vi "Run_Command.vi"(0 "Event":cluster{string, string[], dbl[], dbl}, 1 "Debug Mode":bool, 2 "Realtime Debug":bool, 3 "Update Functions In":cluster{string, string[], dbl[], dbl}[](array[cluster]), 4 "API Function Array":cluster{string, "VI Reference":refnum<vi>}[](array[cluster])) -> (5 "Update Functions Out":cluster{string, string[], dbl[], dbl}[](array[cluster]), 6 "Status Array":cluster{string[], "Status Out":string}[](array[cluster]))   [LabVIEW 2011]
doc: "This VI executes a discrete command given by the \"Event\" parameter. It will also be added to the \"Update Functions\" array if the command needs to be periodically updated as the sequence progresses. \"Debug Mode\" disables all hardware communication and disregards all time values for commands. If \"Realtime Debug\" is also enabled along with \"Debug Mode\", hardware communications will still be disabled but the sequence will proceed with appropriate timing values."
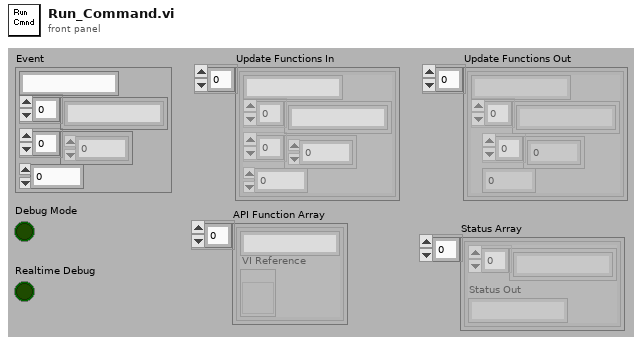
[diagram p1: front panel]
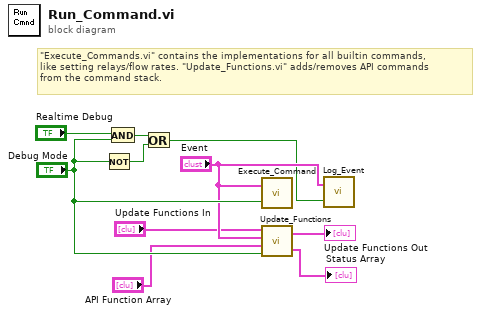
[diagram p0: block diagram]
diagram:
  # "\"Execute_Commands.vi\" contains the implementations for all builtin commands,\nlike setting relays/flow rates. \"Update_Functions.vi\" adds/removes API commands\nfrom the command stack."
  n1 = Not(x="Debug Mode") -> (.not. x?=w9:bool)
  n2 = And(x="Realtime Debug", y="Debug Mode") -> (x .and. y?=w8:bool)
  n3 = Or(x=w8, y=w9) -> (x .or. y?=w3:bool)
  n4 = call "Execute_Command.vi"("Debug"="Debug Mode", "Event"="Event") -> ()  [unwired: 1 out]
  n5 = call "Update_Functions.vi"("Debug"="Debug Mode", "API Function Array"="API Function Array", "Event"="Event", "Update Functions In"="Update Functions In") -> ("Status Array"=→"Status Array":cluster{string[], "Status Out":string}[], "Update Functions Out"=→"Update Functions Out":cluster{string, string[], dbl[], dbl}[])
  n6 = call "Log_Event.vi"("Debug"=w3, "Event"="Event") -> ()  [unwired: 1 out]
